vi "GLDL Update Display.vi"(8 "error in (no error)":errorcluster, 10 "Message Data":variant, 11 "Data Cluster in":T1={"Data Display"="", "FP Control Refs"={"Connect to Station Ref"=refnum, "Download Ref"=refnum, "Exit Button Ref"=refnum, "Start Date Refnum"=refnum, "End Date Refnum"=refnum, "Path"=refnum, "COM Port"="", "IP or Phone Ref"=refnum, "TCPIP ID"=refnum, "Reboot Refnum"=refnum, "Datafile Refnum"=refnum}, "FP Indicator Refs"={"Connected Refnum"=refnum, "Data Display Ref"=refnum, "Station ID Ref"=refnum}, "User Events"={"Stop"=refnum, "Update Display"=refnum}, "Message Queues"={"UI"=refnum, "ACQUISITION"=refnum, "PROCESSING"=refnum, "LOGGING"=refnum}, "IS IP?"=FALSE, "Downloading?"=FALSE, "DCP Version"=enum."XPert2", "Processing Loop State"=enum."Get Station  ID", "Username"=refnum, "Password"=refnum}) -> (0 "error out":errorcluster, 3 "Data Cluster out":T1={"Data Display"="", "FP Control Refs"={"Connect to Station Ref"=refnum, "Download Ref"=refnum, "Exit Button Ref"=refnum, "Start Date Refnum"=refnum, "End Date Refnum"=refnum, "Path"=refnum, "COM Port"="", "IP or Phone Ref"=refnum, "TCPIP ID"=refnum, "Reboot Refnum"=refnum, "Datafile Refnum"=refnum}, "FP Indicator Refs"={"Connected Refnum"=refnum, "Data Display Ref"=refnum, "Station ID Ref"=refnum}, "User Events"={"Stop"=refnum, "Update Display"=refnum}, "Message Queues"={"UI"=refnum, "ACQUISITION"=refnum, "PROCESSING"=refnum, "LOGGING"=refnum}, "IS IP?"=FALSE, "Downloading?"=FALSE, "DCP Version"=enum."XPert2", "Processing Loop State"=enum."Get Station  ID", "Username"=refnum, "Password"=refnum})   [LabVIEW 2018]
uses:
  controls/GLDL UI Data.ctl
  controls/Disconnect Control.ctl
  controls/Download Control.ctl
  controls/Exit Control.ctl
  controls/Date Control.ctl
  controls/IP Phone Number Control.ctl
  controls/Reboot Control.ctl
  controls/Connected Indicator.ctl
  controls/Output Indicator.ctl
  controls/Station ID Indicator.ctl
  Message Queue/All Message Queues.ctl
  Message Queue/Message Cluster.ctl
  controls/Processing Loop State.ctl
  Message Queue/GLDL Message Queue.lvlib
types:
  T1 = typedef "GLDL UI Data.ctl" = cluster{"Data Display":string, "FP Control Refs":cluster{"Connect to Station Ref":refnum<vi>, "Download Ref":refnum<vi>, "Exit Button Ref":refnum<vi>, "Start Date Refnum":refnum<vi>, "End Date Refnum":refnum<vi>, "Path":refnum<vi>, "COM Port":refnum<visa-resource-name>, "IP or Phone Ref":refnum<vi>, "TCPIP ID":refnum<k5>, "Reboot Refnum":refnum<vi>, "Datafile Refnum":refnum<file>}, "FP Indicator Refs":cluster{"Connected Refnum":refnum<vi>, "Data Display Ref":refnum<vi>, "Station ID Ref":refnum<vi>}, "User Events":cluster{"Stop":refnum<user-event>, "Update Display":refnum<user-event>}, "Message Queues":T2, "IS IP?":bool, "Downloading?":bool, "DCP Version":enum16{"XPert", "XPert2"}, "Processing Loop State":T3, "Username":refnum<vi>, "Password":refnum<vi>}
  T2 = typedef "GLDL Message Queue.lvlib/All Message Queues.ctl" = cluster{"UI":refnum<queue>, "ACQUISITION":refnum<queue>, "PROCESSING":refnum<queue>, "LOGGING":refnum<queue>}
  T3 = typedef "Processing Loop State.ctl" = enum16{"Get Station  ID", "Change Directory SD Card", "Change Directory Storage Card", "Downloading", "Idle in DL Directory"}
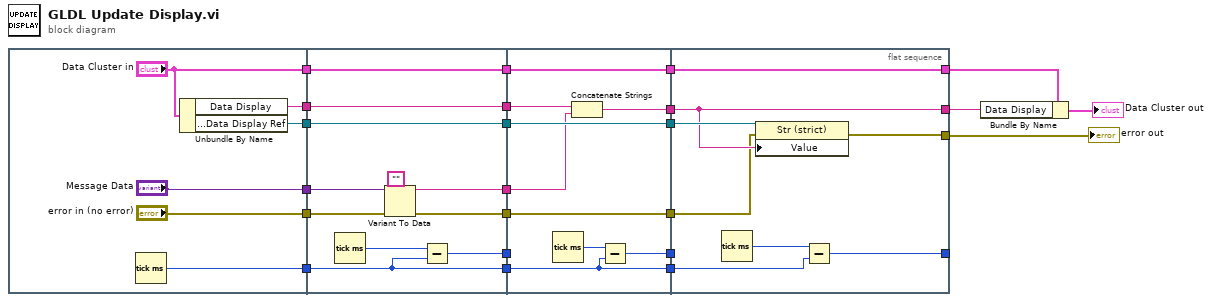
[diagram p0: block diagram]
diagram:
  n1 = flat-sequence {
    tunnel: ["Data Cluster in"] -> w23
    tunnel: [w28] -> w22
    tunnel: ["Message Data"] -> w21
    tunnel: ["error in (no error)"] -> w20
    tunnel: [w25] -> w19
    tunnel: [w24] -> w18
    tunnel: w23 -> [w40]
    tunnel: w22 -> [w30]
    tunnel: w21 -> [w38]
    tunnel: w20 -> [w37]
    tunnel: w19 -> [w31]
    tunnel: w18 -> [w33]
    tunnel: [w40] -> w17
    tunnel: [w31] -> w16
    tunnel: [w33] -> w15
    tunnel: [w36] -> w14
    tunnel: [w35] -> w13
    tunnel: [w32] -> w6
    tunnel: [w30] -> w1
    tunnel: w17 -> [w49]
    tunnel: w16 -> [w48]
    tunnel: w15 -> [w42]
    tunnel: w14 -> [w45]
    tunnel: w13 -> [w47]
    tunnel: [w49] -> w12
    tunnel: [w44] -> w11
    tunnel: [w48] -> w10
    tunnel: [w42] -> w9
    tunnel: [w47] -> w8
    tunnel: w6 -> [_]
    tunnel: [w41] -> w5
    tunnel: w1 -> [w46]
    tunnel: w12 -> [w57]
    tunnel: w11 -> [w55]
    tunnel: w10 -> [w56]
    tunnel: w9 -> [w53]
    tunnel: w8 -> [w52]
    tunnel: w5 -> [_]
    tunnel: [w57] -> w3
    tunnel: [w55] -> w4
    tunnel: [w51] -> w7
    tunnel: [w50] -> _
    frame #0 {
      n2 = Tick Count (ms)() -> (millisecond timer value=w24:u32)
      n3 = Unbundle By Name("Data Cluster in") -> ("Data Display"=w28:string, "FP Indicator Refs.Data Display Ref"=w25:refnum<vi>)
    }
    frame #1 {
      n4 = Tick Count (ms)() -> (millisecond timer value=w34:u32)
      n5 = Variant To Data(error in=w37, type="", Variant=w38) -> (data=w36:string, error out=w35:errorcluster)
      n6 = Subtract(x=w34, y=w33) -> (x-y=w32:u32)
    }
    frame #2 {
      n7 = Tick Count (ms)() -> (millisecond timer value=w43:u32)
      n8 = Concatenate Strings(w46, w45) -> (w44:string)
      n9 = Subtract(x=w43, y=w42) -> (x-y=w41:u32)
    }
    frame #3 {
      n10 = Tick Count (ms)() -> (millisecond timer value=w54:u32)
      n11 = property class="Str (strict)"(reference=w56, error in=w52, "Value"=w55) -> (error out=w51:errorcluster)  [unwired: 1 out]
      n12 = Subtract(x=w54, y=w53) -> (x-y=w50:u32)
    }
  }
  n13 = Bundle By Name(cluster=w3, "Data Display"=w4) -> (→"Data Cluster out":T1)
  "error out" <- w7
